vi "Write Array ref value.vi"(8 "Error In":errorcluster, 10 "Array":refnum<class "Subpanel Inserter.lvclass">[](array[class]), 11 "Generic Prompt.lvclass":refnum<class "Generic Prompt.lvclass">) -> (0 "Error Out":errorcluster, 3 "Generic Prompt.lvclass 2":refnum<class "Generic Prompt.lvclass">)   [LabVIEW 2016, in "Generic Prompt.lvlib" / "Generic Prompt.lvclass"]
uses:
  Generic Prompt.lvclass
  Subpanel Insertion/Subpanel Inserter.lvclass
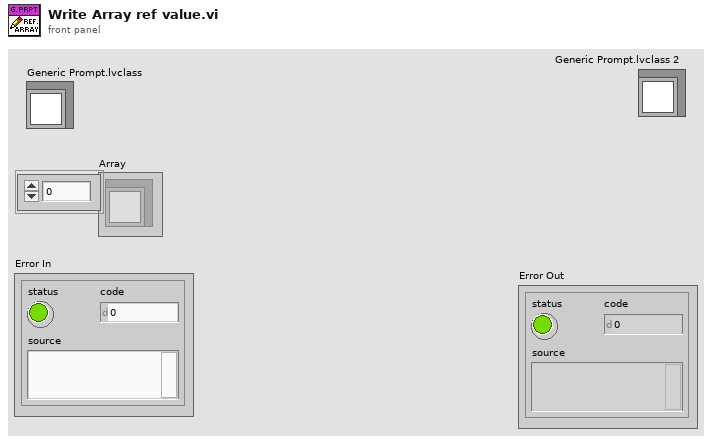
[diagram p1: front panel]
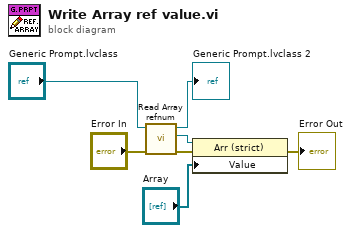
[diagram p0: block diagram]
diagram:
  n1 = call-dynamic "Read Array refnum.vi"("error in (no error)"="Error In", "Generic Prompt in"="Generic Prompt.lvclass") -> ("error out"=w3:errorcluster, "Array refnum"=w5:refnum<vi>, "Generic Prompt out"=→"Generic Prompt.lvclass 2":refnum<class "Generic Prompt.lvclass">)  [unwired: 7 in]
  n2 = property class="Arr (strict)"(reference=w5, error in=w3, "Value"="Array") -> (error out=→"Error Out":errorcluster)  [unwired: 1 out]
